vi "lxw parse cell.vi"(8 "error in (no error)":errorcluster, 9 "col":u16, 10 "row":u32, 11 "cell_str":string) -> (0 "error out":errorcluster, 1 "col out":u16, 2 "row out":u32)   [LabVIEW 2015, in "xlsxwriter.lvlib"]
doc: "void lxw_parse_cell(const char *cell_str, lxw_row_t *row, lxw_col_t *col);"
uses:
  xlsxwriter.lvlib
  xlsxwriter.dll
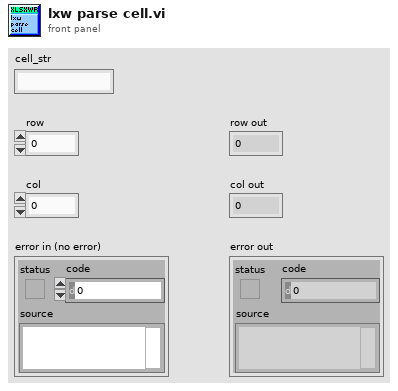
[diagram p1: front panel]
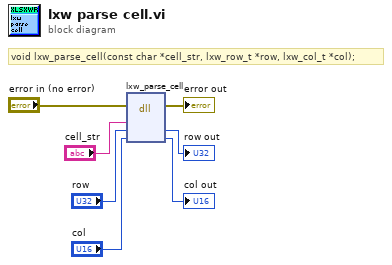
[diagram p0: block diagram]
diagram:
  # "void lxw_parse_cell(const char *cell_str, lxw_row_t *row, lxw_col_t *col);"
  n1 = dll-call lib="C:/Users/WDAGUtilityAccount/Desktop/lv_vis_added_cell/xlsxwriter.*" fn="lxw_parse_cell"(error in="error in (no error)", "cell_str"="cell_str", "row"="row", "col"="col") -> (error out=→"error out":errorcluster, "row"=→"row out":u32, "col"=→"col out":u16)  [unwired: 4 in, 1 out]
